vi "Read Temperature Chamber.vi"() -> (1 "Floor Temperature":dbl, 2 "Door Temperature":dbl, 3 "Ceiling Temperature":dbl)   [LabVIEW 2020]
uses:
  <vilib>/gmath/statdist.llb/Normal Random.vi
  <vilib>/gmath/NI_Gmath.lvlib
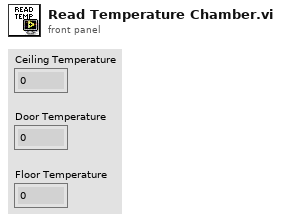
[diagram p1: front panel]
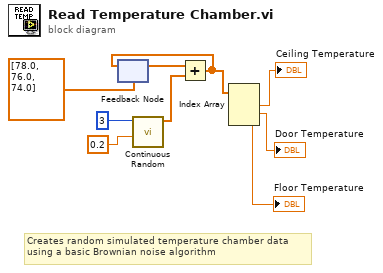
[diagram p0: block diagram]
diagram:
  # "Creates random simulated temperature chamber data\nusing a basic Brownian noise algorithm"
  n1 = feedback #1(dbl[] [78.0, 76.0, 74.0]) -> (w9:dbl[])
  n2 = call-poly <vilib>:"Continuous Random.vi"("std"=0.2, "samples"=3) -> ("normal random data"=w5:dbl[])  [unwired: 8 in, 1 out]
  n3 = Add(x=w9, y=w5) -> (x+y=w4:dbl[])
  n4 = feedback-in #1(w4) -> ()
  n5 = Index Array(array=w4) -> (element #1=→"Ceiling Temperature":dbl, element #2=→"Door Temperature":dbl, element #3=→"Floor Temperature":dbl)  [unwired: 3 in]
